vi "Alazar_simulate.vi"(7 "Enum":enum16{"init", "output"}(ring)=enum."output") -> (3 "Array":u16[](array[numeric]))   [LabVIEW 2018]
uses:
  Controls/FGV Actions.ctl
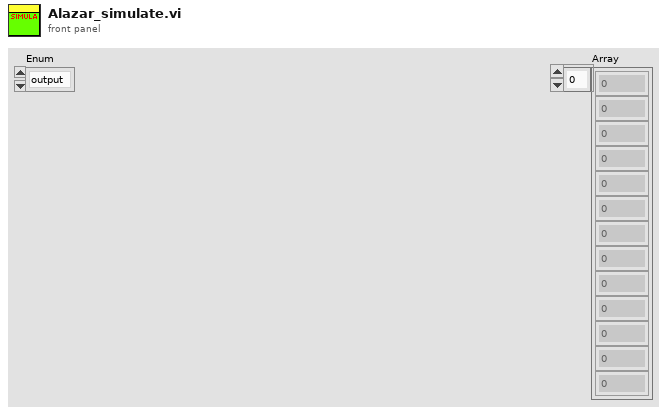
[diagram p1: front panel]
types:
  T1 = typedef "FGV Actions.ctl" = enum16{"Init", "Set", "Get", "Clear"}
  T2 = typedef "System Parameters.ctl" = cluster{"Optical Parameters":T3, "Vibratome":T4, "Table Stages":T5, "Imaging Parameter":T8, "Galvo HW Parameters":cluster{"Analog Out Channel":tag, "Min Voltage":dbl, "Max Voltage":dbl, "Pixel Clock Source":tag, "Sample Rate":dbl, "Line Clock Out Ch":tag}, "Alazar parameters":T10, "Mosaic Paramter":cluster{"X Axis":cluster{"Start [mm]":dbl, "Steps [pts]":dbl, "End [mm]":dbl}, "Y Axis":cluster{"Start [mm]":dbl, "Steps [pts]":dbl, "End [mm]":dbl}, "Scan Pattern":enum16{"Uni-directional", "Bi-Directional", "Spiral Out", "Spiral In"}, "Overlap Options":cluster{"Overlap Type":enum16{"No Overlap", "X Only", "Y Only", "X and Y"}, "Percent Overlap":u8, "Justify":enum16{"Start", "Center", "End"}}}, "Manual Controls":T17, "Vibratome Axis":T20}
  T3 = typedef "Optical Parameters.ctl" = cluster{"Obj. Focal Length [mm]":dbl, "Scan Lens EFL[mm]":dbl, "Tube Lens EFL[mm]":dbl, "Galvo V Range (+/-)":dbl, "Galvo Max Half Angle [Deg]":dbl, "Max Galvo Range[%]":dbl}
  T4 = typedef "Vibratome Parameters.ctl" = cluster{"Z Bottom [mm]":dbl, "Pre Cut Dwell [s]":dbl, "Blade Frequency [RPM]":u16, "Slice Speed [mm/s]":dbl, "Post Cut Dwell [s]":dbl, "Ramp Time [s]":dbl, "Start X [mm]":dbl, "Start Y [mm]":dbl, "Slice Length [mm]":dbl, "Slice Axis":enum16{"X Axis", "Y Axis", "Z Axis"}, "Controller VISA Ref":refnum<visa-resource-name>, "Blade Frequency [Hz]":u16, "Analog Out Channel":tag, "Pixel Clock Source":tag}
  T5 = typedef "Translation Stage Parameters.ctl" = cluster{"X Stage":T6, "Y Stage":T6, "Z Stage":T6}
  T6 = typedef "Translation Stage Cluster.ctl" = cluster{"Position":dbl, "Is.Enabled?":bool, "Is.Connected?":bool, "Device SN":string, "AccelerationMaximum":dbl, "VelocityMaximum":dbl, "Acceleration":dbl, "Velocity":dbl, "waitTimeout (ms)":i32, "Model":T7, "Is.Homed?":bool, "MOVE":bool}
  T7 = typedef "Translation Stage Types.ctl" = enum16{"None", "Thorlabs LTS", "Thorlabs MLJ"}
  T8 = typedef "Imaging Parameters.ctl" = cluster{"Raster Scan Direction":T9, "Pixel Dwell Time [Clock Cycles]":u16, "Flyback Time [Clock Cycles]":u16, "XY Center [um]":cluster{"X":dbl, "Y":dbl}, "Pixel Step Size [um] X":dbl, "XY Image Size":enum16{"32 x 32", "64 x 64", "128 x 128", "256 x 256", "512 x 512", "1024 x 1024", "2048 x 2048"}, "Custom":bool, "Custom Size":cluster{"X":u16, "Y":u16}, "Line Averages":u8, "Pixel Step Size [um] Y":dbl}
  T9 = typedef "Scan Direction.ctl" = enum16{"Uni Directional", "Bi Directional", "None"}
  T10 = typedef "Alazar parameters.ctl" = cluster{"Trigger Settings":cluster{"General Trigger Settings":T11, "Trigger Engine 1":T12, "Trigger Engine 2":T12}, "Device ID":T13, "Ch A Input Control":T14, "Ch B Input Control":T14, "Acq Settings":T15, "Capture Clock":T16}
  T11 = typedef "General Trigger Settings.ctl" = cluster{"Trigger Operation":u32, "Coupling ID":u32, "Range ID":u32, "Delay":u32, "Timeout Ticks":u32, "Mode":u32, "Parameter":u32}
  T12 = typedef "Trigger Engine Controls.ctl" = cluster{"Trigger Engine":u32, "Source":u32, "Slope":u32, "Level":u32}
  T13 = typedef "Alazar Device ID.ctl" = cluster{"System ID":u32, "Board ID":u32}
  T14 = typedef "Channel Input Controls.ctl" = cluster{"Channel":u8, "Coupling":u32, "Range":u32, "Impedance":u32}
  T15 = typedef "Alazar Acquisition Settings.ctl" = cluster{"Record Length":u32, "Offset":u32, "Records Per Buffer":u32, "Records Count (Records/Acq)":u32, "Window Type":u32, "Footer":u32, "Samples per record":u32, "Output Format":u32}
  T16 = typedef "Clock Controls.ctl" = cluster{"Sample Rate":u32, "Decimation":u32, "Source":u32, "Edge":u32}
  T17 = typedef "Manual Controls.ctl" = cluster{"Z0":dbl, "First image height":dbl, "Data Path":path, "Save parameters":T18, "Center Galvos":bool, "Acquisition mode":T19, "PSOCT Channel":u32, "Save":bool, "AIP rotation angle":dbl, "Scan Parameters":cluster{"# Scan":cluster{"#Ascan":i32, "#Bscan":i32}, "# Rpt":cluster{"#ARpt":i32, "#BRpt":i32}, "Aline Rate":u16, "# Extra":cluster{"# ARpt_extra":i32, "#Brtn_extra":i32}}, "ROI Parameters":cluster{"ROI (mm)":cluster{"X (mm)":dbl, "Y (mm)":dbl}, "Shift (mm)":cluster{"Xshift (mm)":sgl, "Yshift (mm)":sgl}}, "Objective":u16, "ret ds":bool, "Pause?":bool, "Outgoing Mail Server (SMTP)":string, "Email":string, "Password":string, "Carrier":enum16{"T-Mobile", "AT&T", "Verizon", "Sprint"}, "phone number":string, "Subject":string, "Message":string, "blocker position":enum16{"every two slices", "Nat slices", "None"}}
  T18 = typedef "FFT parameters.ctl" = cluster{"start pixel":i32, "#pixels to save":i32}
  T19 = typedef "FFT mode.ctl" = enum16{"ThorOCT B line", "ThorOCT Spectral", "ThorOCT FFT", "Alazar B line", "Alazar FFT", "GPU FFT", "Alazar Spectral", "Simulation", "auto adjust focus"}
  T20 = typedef "Vibratome Param.ctl" = cluster{"Start [mm](first cut height)":dbl, "slice thickness[um]":dbl, "#slice":u16, "image thickness(um)":dbl, "#images":u16, "30um?":bool}
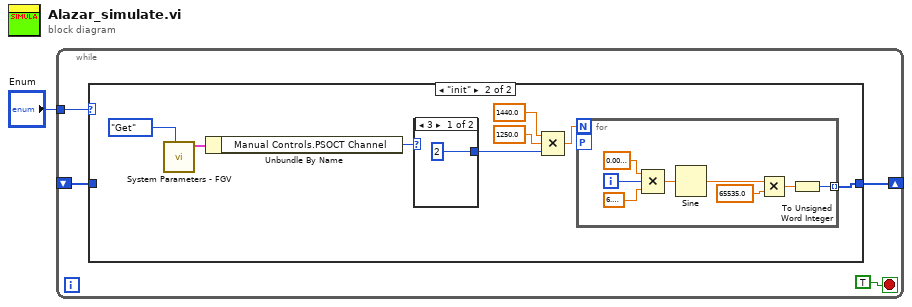
[diagram p0: block diagram]
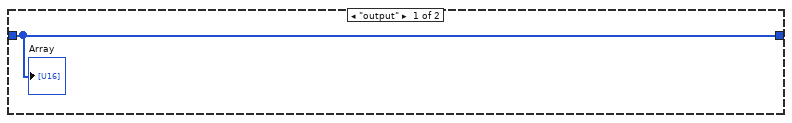
[diagram p2: hidden frame]
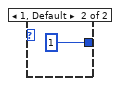
[diagram p3: hidden frame]
diagram:
  n1 = while {
    tunnel: "Enum" -> [w4]
    shift-right: [w2] -> _
    shift-left: _ -> [w3]
    stop <- TRUE stop-if-true
    n2 = case shown="\"init\"" w4 {
      tunnel: [w6 w7] -> w2
      tunnel: w3 -> [w6 _]
      frame "output" {
        "Array" <- w6
      }
      frame "init" {
        n3 = call "System Parameters - FGV.vi"("Actions"=FGV_Actions."Get") -> ("System Parameters [Out]"=w10:T2)  [unwired: 9 in, 1 out]
        n4 = Unbundle By Name(w10) -> ("Manual Controls.PSOCT Channel"=w9:u32)
        n5 = case shown="3" w9 {
          tunnel: [2 1] -> w8
          frame 3 {
          }
          frame 1, Default {
          }
        }
        n6 = Compound Arithmetic op=MULTIPLY(1440.0 ("x"), 1250.0 ("y"), w8) -> (w11:dbl)
        n7 = for {
          N: w11 -> [_]
          tunnel: [w24] -> w7 mode=indexing
          workers-P: _ -> [_]
          i -> [w18]
          n8 = Compound Arithmetic op=MULTIPLY(sgl 0.01 ("x"), w18, 6.283185307179586) -> (w20:dbl)
          n9 = Sine(x=w20) -> (sin(x)=w23:dbl)
          n10 = Multiply(x=w23, y=sgl 65535.0) -> (x*y=w21:dbl)
          n11 = To Unsigned Word Integer(number=w21) -> (unsigned 16bit integer=w24:u16)
        }
      }
    }
  }
